vi "Read.vi"(8 "error in (no error)":errorcluster, 11 "VGC in":refnum<class "PL Inficon VGC.lvclass">) -> (0 "error out":errorcluster, 2 "read buffer":string, 3 "VGC out":refnum<class "PL Inficon VGC.lvclass">)   [LabVIEW 2015, in "PL Inficon VGC.lvclass"]
doc: "Reads bytes from specified interface."
uses:
  PL Inficon VGC.lvclass
  PL Inficon VGC.lvclass/PL Inficon VGC.ctl
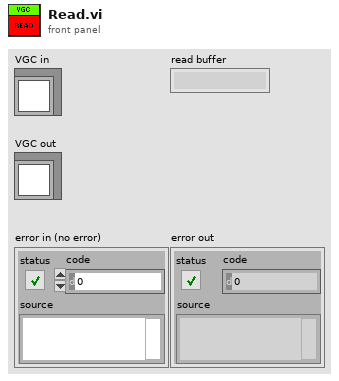
[diagram p1: front panel]
types:
  T1 = enum16{"Standard", "Buffered", "CRLF", "Immediate"}
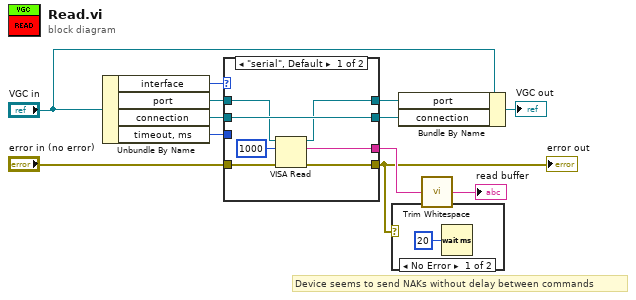
[diagram p0: block diagram]
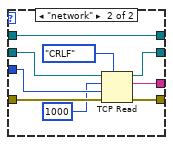
[diagram p3: hidden frame]
diagram:
  # "Device seems to send NAKs without delay between commands"
  n1 = Unbundle By Name("VGC in") -> ("interface"=w11:enum16{"serial", "network"}, "port"=w10:refnum<visa-resource-name>, "connection"=w9:refnum<k5>, "timeout, ms"=w8:u32)
  n2 = case shown="\"serial\", Default" w11 {
    tunnel: "error in (no error)" -> [w17 w27]
    tunnel: [w15 w28] -> w1
    tunnel: w10 -> [w18 w25]
    tunnel: w9 -> [w19 w26]
    tunnel: [w14 w25] -> w6
    tunnel: w8 -> [_ w24]
    tunnel: [w19 w23] -> w5
    tunnel: [w13 w20] -> w3
    frame "serial", Default {
      n3 = VISA Read(VISA resource name=w18, byte count=u32 1000, error in (no error)=w17) -> (VISA resource name out=w14:refnum<visa-resource-name>, read buffer=w13:string, error out=w15:errorcluster)  [unwired: 1 out]
    }
    frame "network" {
      n4 = TCP Read(connection ID=w26, bytes to read=1000, error in (no error)=w27, 7:T1."CRLF" ("mode (standard)"), 9:w24) -> (connection ID out=w23:refnum<k5>, data out=w20:string, error out=w28:errorcluster)
    }
  }
  "error out" <- w1
  n5 = case shown="No Error" w1 {
    frame No Error {
      n6 = Wait (ms)(milliseconds to wait=u32 20) -> ()  [unwired: 1 out]
    }
    frame Error {
    }
  }
  n7 = Bundle By Name(cluster="VGC in", "port"=w6, "connection"=w5) -> (→"VGC out":refnum<class "PL Inficon VGC.lvclass">)
  n8 = call <vilib>:"Trim Whitespace.vi"("string"=w3) -> ("trimmed string"=→"read buffer":string)  [unwired: 1 in]
